vi "Playback_gauss2_fitting_Aug14_2016.vi"() -> ()   [LabVIEW 2015]
panel:
  out "Filename 2":path=path "Fitting_Aug15_2016/RawData_Fly1035_E1_M_2015Nov9.tdms" caption="Filename"
  in  "Filename":path=path "Fitting_Aug15_2016/RawData_Fly1035_E1_M_2015Nov9.tdms"
  out "data":string
  out "error out 2":errorcluster
  out "Filename Out":path
  out "error out":errorcluster
  out "Signals 2":dbl
  out "Signals":dynamicdata(graph)
  out "Numeric":i32
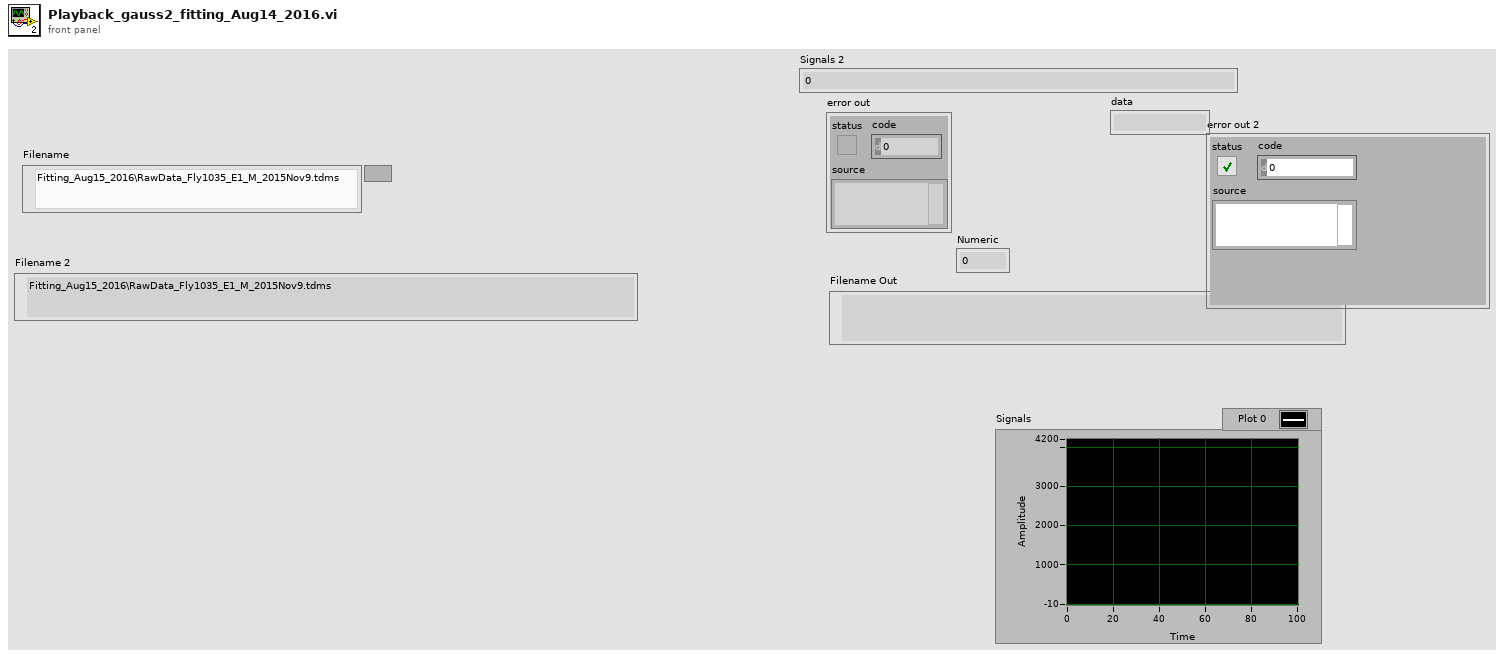
[diagram p1: front panel]
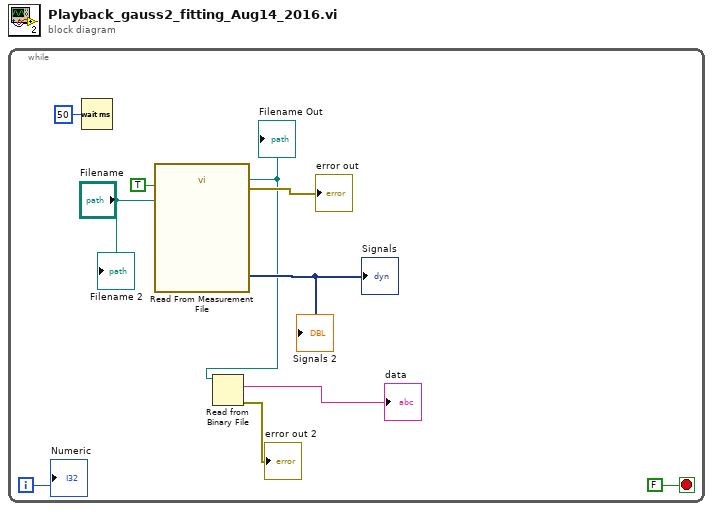
[diagram p0: block diagram]
diagram:
  n1 = while {
    i -> [w9]
    stop <- FALSE stop-if-true
    n2 = Wait (ms)(milliseconds to wait=u32 50) -> ()  [unwired: 1 out]
    n3 = call "Read From Measurement File"("Filename"="Filename", "Enable"=TRUE) -> ("error out"=→"error out":errorcluster, "Filename Out"=w4:path, "Signals"=→"Signals" →"Signals 2":dynamicdata)  [unwired: 4 in, 3 out]
    "Filename Out" <- w4
    n4 = Read from Binary File(11:w4) -> (0:→"error out 2":errorcluster, 2:→"data":string)  [unwired: 5 in, 2 out]
    "Numeric" <- w9
    "Filename 2" <- "Filename"
  }
